vi "Filter.vi"(10 "Output 1":u8[][](array[numeric]), 11 "Filters":T1(ring)) -> (3 "Filtered X":dbl[][](array[numeric]))   [LabVIEW 2016]
uses:
  <vilib>/Analysis/3filter.llb/Equi-Ripple LowPass (DBL).vi
  <vilib>/Analysis/3filter.llb/Equi-Ripple HighPass (DBL).vi
  <vilib>/Analysis/3filter.llb/Equi-Ripple BandPass (DBL).vi
  <vilib>/Analysis/3filter.llb/Equi-Ripple BandStop (DBL).vi
  <vilib>/Analysis/3filter.llb/Butterworth Filter (DBL).vi
  <vilib>/Analysis/NI_AALBase.lvlib
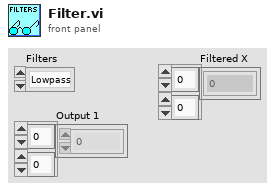
[diagram p1: front panel]
types:
  T1 = enum32{"Lowpass ", "Highpass", "Band pass", "Band Stop", "Butter Worth "}
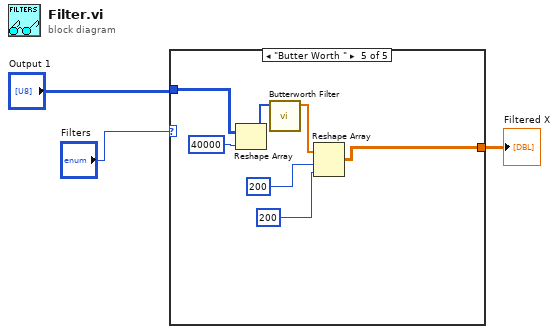
[diagram p0: block diagram]
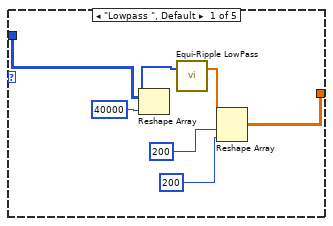
[diagram p2: hidden frame]
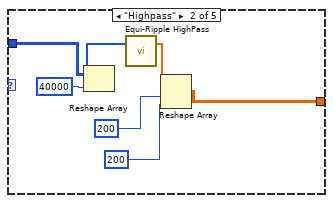
[diagram p3: hidden frame]
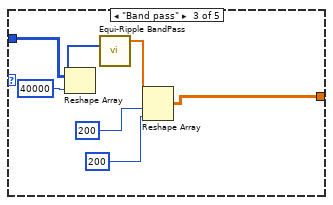
[diagram p4: hidden frame]
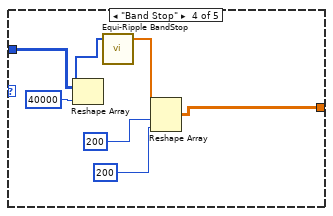
[diagram p5: hidden frame]
diagram:
  n1 = case shown="\"Butter Worth \"" "Filters" {
    tunnel: "Output 1" -> [w5 w16 w21 w28 w35]
    tunnel: [w4 w11 w18 w27 w32] -> w3
    frame "Lowpass ", Default {
      n2 = Reshape Array(w5, 40000 ("dimension size")) -> (w7:u8[])
      n3 = call-poly <vilib>:"Equi-Ripple LowPass.vi"("X"=w7) -> ("Filtered X"=w6:dbl[])  [unwired: 5 in, 1 out]
      n4 = Reshape Array(w6, 200 ("dimension size"), 200 ("dimension size")) -> (w4:dbl[][])
    }
    frame "Highpass" {
      n5 = Reshape Array(w16, 40000 ("dimension size")) -> (w15:u8[])
      n6 = call-poly <vilib>:"Equi-Ripple HighPass.vi"("X"=w15) -> ("Filtered X"=w14:dbl[])  [unwired: 5 in, 1 out]
      n7 = Reshape Array(w14, 200 ("dimension size"), 200 ("dimension size")) -> (w11:dbl[][])
    }
    frame "Band pass" {
      n8 = Reshape Array(w21, 40000 ("dimension size")) -> (w20:u8[])
      n9 = call-poly <vilib>:"Equi-Ripple BandPass.vi"("X"=w20) -> ("Filtered X"=w19:dbl[])  [unwired: 7 in, 1 out]
      n10 = Reshape Array(w19, 200 ("dimension size"), 200 ("dimension size")) -> (w18:dbl[][])
    }
    frame "Band Stop" {
      n11 = Reshape Array(w28, 40000 ("dimension size")) -> (w26:u8[])
      n12 = call-poly <vilib>:"Equi-Ripple BandStop.vi"("X"=w26) -> ("Filtered X"=w25:dbl[])  [unwired: 7 in, 1 out]
      n13 = Reshape Array(w25, 200 ("dimension size"), 200 ("dimension size")) -> (w27:dbl[][])
    }
    frame "Butter Worth " {
      n14 = Reshape Array(w35, 40000 ("dimension size")) -> (w34:u8[])
      n15 = call-poly <vilib>:"Butterworth Filter.vi"("X"=w34) -> ("Filtered X"=w33:dbl[])  [unwired: 7 in, 1 out]
      n16 = Reshape Array(w33, 200 ("dimension size"), 200 ("dimension size")) -> (w32:dbl[][])
    }
  }
  "Filtered X" <- w3
